vi "MatchYear.vi"(6 "Freshmen Graduating Year":i8, 8 "Error In":errorcluster, 9 "Student Counter Per Year":i32[](array[numeric]), 10 "Student Email List":string, 11 "Starting # of Students":i32) -> (0 "Error Out":errorcluster, 1 "Student Counter Per Year":i32[](array[numeric]), 2 "Match Found?":bool, 3 "Number of Students Found":i32)   [LabVIEW 2015]
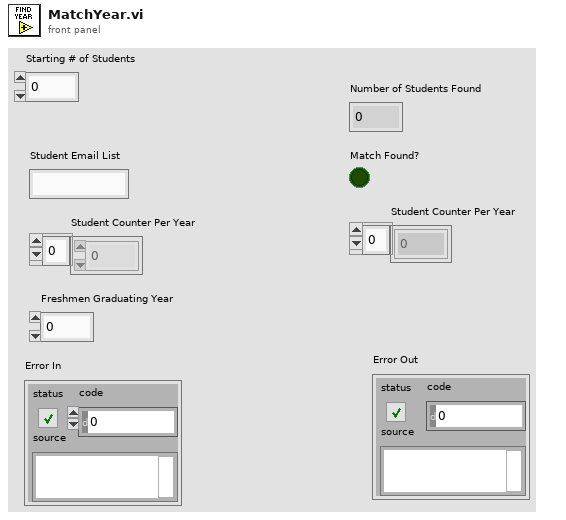
[diagram p1: front panel]
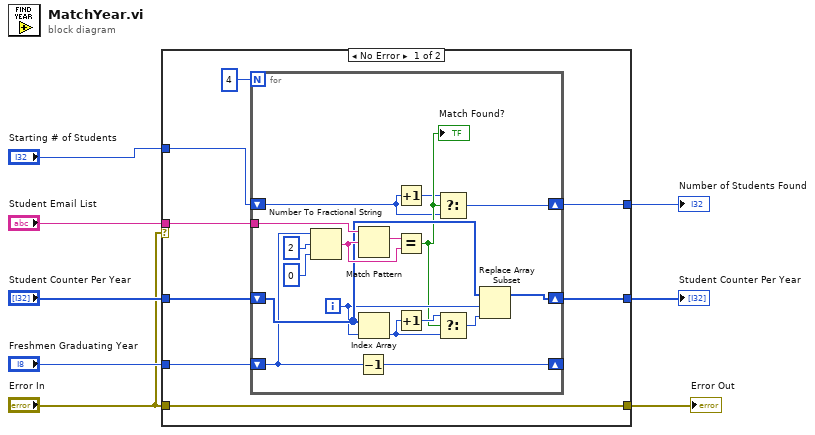
[diagram p0: block diagram]
diagram:
  n1 = case shown="No Error" "Error In" {
    tunnel: [w16 w34] -> w8
    tunnel: "Starting # of Students" -> [w15 w34]
    tunnel: [w14 w35] -> w6
    tunnel: "Student Counter Per Year" -> [w13 w35]
    tunnel: "Freshmen Graduating Year" -> [w11 _]
    tunnel: "Student Email List" -> [w10 _]
    tunnel: [w9 w36] -> w2
    tunnel: "Error In" -> [w9 w36]
    frame No Error {
      n2 = for {
        N: 4 -> [_]
        tunnel: w10 -> [w33]
        shift-right: [w23] -> w14
        shift-left: w13 -> [w27]
        shift-right: [w21] -> _
        shift-left: w11 -> [w22]
        shift-right: [w17] -> w16
        shift-left: w15 -> [w18]
        i -> [w26]
        n3 = Number To Fractional String(number=w22, width (-)=i16 2, precision (6)=i16 0) -> (F-format string=w30:string)  [unwired: 1 in]
        n4 = Decrement(x=w22) -> (x-1=w21:i8)
        n5 = Match Pattern(string=w33, regular expression=w30) -> (match substring=w31:string)  [unwired: 1 in, 3 out]
        n6 = Index Array(array=w27, index=w26) -> (element=w25:i32)
        n7 = Increment(x=w18) -> (x+1=w19:i32)
        n8 = Equal?(x=w31, y=w30) -> (x = y?=w20:bool)
        "Match Found?" <- w20
        n9 = Increment(x=w25) -> (x+1=w29:i32)
        n10 = Select(t=w19, s=w20, f=w18) -> (s? t:f=w17:i32)
        n11 = Select(t=w29, s=w20, f=w25) -> (s? t:f=w24:i32)
        n12 = Replace Array Subset(array=w27, new element=w24, index=w26) -> (w23:i32[])
      }
    }
    frame Error {
    }
  }
  "Number of Students Found" <- w8
  "Student Counter Per Year" <- w6
  "Error Out" <- w2
